vi "ExtractFreeshapeROI.vi"(2 "error out 2":errorcluster, 3 "Image Out":T1) -> (0 "error out":errorcluster, 1 "Image Dst Out":T1)   [LabVIEW 2010]
uses:
  <vilib>/vision/Image Controls.llb/IMAQ Image.ctl
  <vilib>/vision/NI_Vision_Development_Module.lvlib
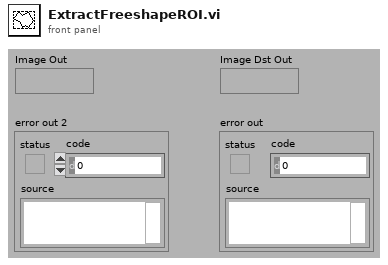
[diagram p1: front panel]
types:
  T1 = typedef "IMAQ Image.ctl" = refnum<image>
  T2 = typedef "Image Type" = u32
  T3 = typedef "ROI Descriptor" = cluster{"Global Rectangle":i32[], "Contours":cluster{"ID":enum32{"External", "Internal"}, "Type":u32, "Coordinates":i32[]}[]}
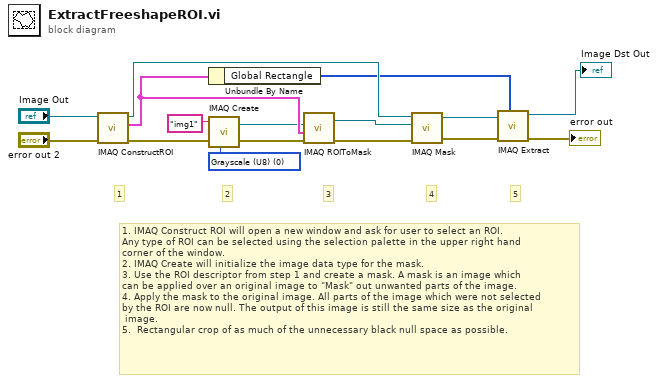
[diagram p0: block diagram]
diagram:
  w2 = T2 0 items=["Grayscale (U8)", "Grayscale (I16)", "Grayscale (SGL)", "Complex (CSG)", "RGB (U32)", "HSL (U32)", "RGB (U64)"] ("Image Type")
  # "1. IMAQ Construct ROI will open a new window and ask for user to select an ROI. \nAny type of ROI can be selected using the selection palette in the upper right hand\ncorner of the window.\n2. IMAQ Create will initialize the image data type for the mask. \n3. Use the ROI descriptor from step 1 and create a mask. A mask is an image which\ncan be applied over an original image to \"Mask\" out unwanted parts of the image.\n4. Apply the mask to the original image. All parts of the image which were not selected\nby the ROI are now null. The output of this image is still the same size as the original\n image. \n5.  Rectangular crop of as much of the unnecessary black null space as possible."
  # "5"
  # "4"
  # "3"
  # "2"
  # "1"
  n1 = call "IMAQ ConstructROI"("error in (no error)"="error out 2", "Image"="Image Out") -> ("error out"=w9:errorcluster, "ROI Descriptor Out"=w5:T3, "Image Out (duplicate)"=w14:T1)  [unwired: 6 in, 1 out]
  n2 = Unbundle By Name(w5) -> ("Global Rectangle"=w6:i32[])
  n3 = call "IMAQ Create"("Image Name"="img1", "Image Type"=w2, "error in (no error)"=w9) -> ("New Image"=w4:T1, "error out"=w10:errorcluster)  [unwired: 2 in]
  n4 = call "IMAQ ROIToMask"("error in (no error)"=w10, "ROI Descriptor"=w5, "Image"=w4) -> ("error out"=w12:errorcluster, "Image Out"=w15:T1)  [unwired: 3 in, 1 out]
  n5 = call "IMAQ Mask"("error in (no error)"=w12, "Image Mask"=w15, "Image Src"=w14) -> ("error out"=w13:errorcluster, "Image Dst Out"=w16:T1)  [unwired: 2 in]
  n6 = call "IMAQ Extract"("Optional Rectangle"=w6, "error in (no error)"=w13, "Image Src"=w16) -> ("error out"=→"error out":errorcluster, "Image Dst Out"=→"Image Dst Out":T1)  [unwired: 7 in]
